vi "convert_string_to_doubleArray.vi"(2 "Max Elements Count (All)":i32=-1, 3 "default (0)":dbl, 4 "string in":string) -> (0 "double array size out":i32 caption="double array size", 1 "double array out":dbl[](array[numeric]))   [LabVIEW 2014, in "rszvl_rsidr_core.lvlib"]
uses:
  rszvl_rsidr_core.lvlib
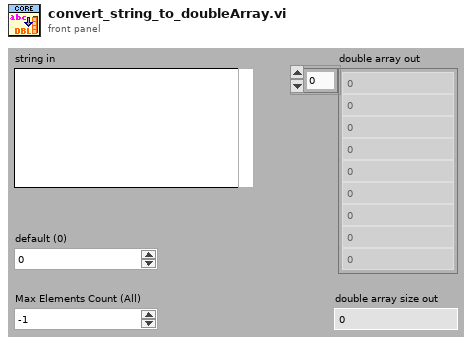
[diagram p1: front panel]
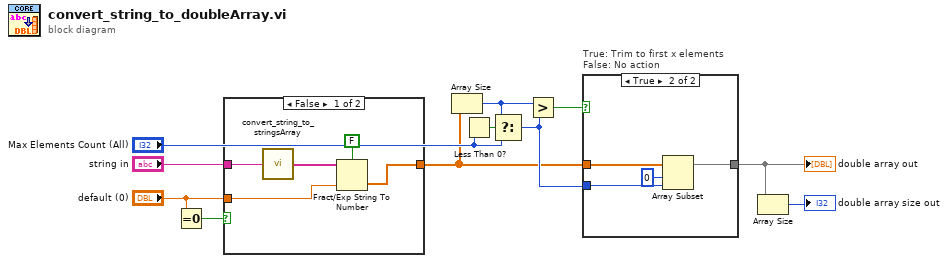
[diagram p0: block diagram]
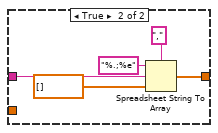
[diagram p3: hidden frame]
diagram:
  n1 = Equal To 0?(x="default (0)") -> (x = 0?=w9:bool)
  n2 = case shown="False" w9 {
    tunnel: "string in" -> [w16 w18]
    tunnel: [w13 w17] -> w2
    tunnel: "default (0)" -> [w12 _]
    frame False {
      n3 = call "convert_string_to_stringsArray.vi"("String in"=w16) -> ("string array out"=w14:string[])  [unwired: 3 in, 1 out]
      n4 = Fract/Exp String To Number(use system decimal point (T)=FALSE, string=w14, default (0 dbl)=w12) -> (number=w13:dbl[])  [unwired: 1 in, 1 out]
    }
    frame True {
      n5 = Spreadsheet String To Array(delimiter (Tab)=",", format string="%.;%e", spreadsheet string=w18, array type (2D Dbl)=dbl[] [] ("List Power Results")) -> (array=w17:dbl[])
    }
  }
  n6 = Array Size(array=w2) -> (size(s)=w6:i32)
  n7 = Less Than 0?(x="Max Elements Count (All)") -> (x < 0?=w7:bool)
  n8 = Select(t=w6, s=w7, f="Max Elements Count (All)") -> (s? t:f=w3:i32)
  n9 = Greater?(x=w6, y=w3) -> (0:w5:bool)
  n10 = case "True: Trim to first x elements\nFalse: No action" shown="True" w5 {
    tunnel: [w22 w23] -> w1
    tunnel: w2 -> [w22 w26]
    tunnel: w3 -> [_ w24]
    frame False {
    }
    frame True {
      n11 = Array Subset(array=w26, index=0, length=w24) -> (w23:dbl[])
    }
  }
  "double array out" <- w1
  n12 = Array Size(array=w1) -> (size(s)=→"double array size out":i32)
